vi "Start.vi"(8 "error in (no error)":errorcluster, 11 "TrialBasedExperiment in":refnum<class "TrialBasedExperiment.lvclass">) -> (0 "error out":errorcluster, 3 "TrialBasedExperiment out":refnum<class "TrialBasedExperiment.lvclass">)   [LabVIEW 2010, in "TrialBasedExperiment.lvclass"]
uses:
  TrialBasedExperiment.lvclass
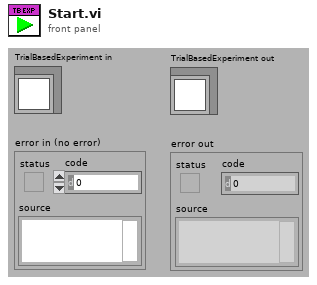
[diagram p1: front panel]
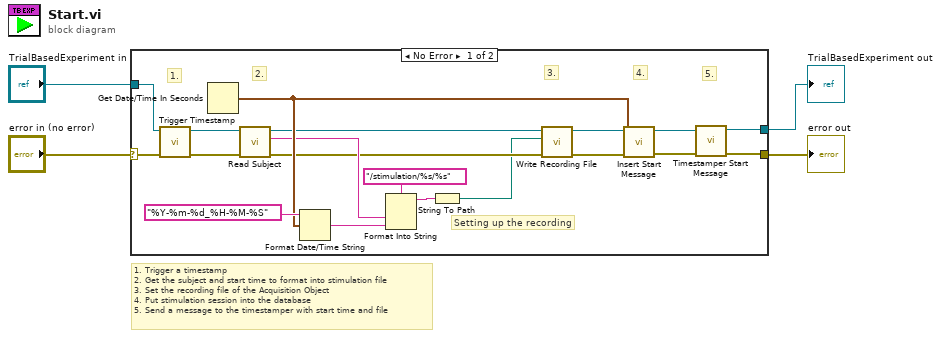
[diagram p0: block diagram]
diagram:
  # "1. Trigger a timestamp\n2. Get the subject and start time to format into stimulation file\n3. Set the recording file of the Acquisition Object\n4. Put stimulation session into the database\n5. Send a message to the timestamper with start time and file"
  n1 = case shown="No Error" "error in (no error)" {
    selector: "error in (no error)" -> [w23 w25]
    tunnel: [w19 w25] -> w3
    tunnel: [w18 w24] -> w1
    tunnel: "TrialBasedExperiment in" -> [w22 w24]
    frame No Error {
      # "5."
      # "4."
      # "3."
      # "2."
      # "1."
      # "Setting up the recording"
      n2 = call-dynamic "Trigger Timestamp.vi"("error in (no error)"=w23, "TrialBasedExperiment in"=w22) -> ("error out"=w12:errorcluster, "TrialBasedExperiment out"=w13:refnum<class "TrialBasedExperiment.lvclass">)  [unwired: 8 in]
      n3 = Get Date/Time In Seconds() -> (seconds since 1Jan1904=w16:timestamp)
      n4 = call-dynamic "Read Subject.vi"("error in (no error)"=w12, "TrialBasedExperiment in"=w13) -> ("error out"=w9:errorcluster, "Subject"=w11:string, "TrialBasedExperiment out"=w10:refnum<class "TrialBasedExperiment.lvclass">)  [unwired: 7 in]
      n5 = Format Date/Time String(time format string (%c)="%Y-%m-%d_%H-%M-%S", seconds (now)=w16) -> (date/time string=w14:string)  [unwired: 1 in]
      n6 = Format Into String(format string="/stimulation/%s/%s", w11, w14) -> (resulting string=w6:string)  [unwired: 2 in, 1 out]
      n7 = String To Path(string=w6) -> (path=w5:path)
      n8 = call-dynamic "Write Recording File.vi"("error in (no error)"=w9, "Recording File"=w5, "AcquistionObject in"=w10) -> ("error out"=w7:errorcluster, "AcquistionObject out"=w8:refnum<class "TrialBasedExperiment.lvclass">)  [unwired: 7 in]
      n9 = call-dynamic "Insert Start Message.vi"("error in (no error)"=w7, "Start Time"=w16, "TrialBasedExperiment in"=w8) -> ("error out"=w20:errorcluster, "TrialBasedExperiment out"=w21:refnum<class "TrialBasedExperiment.lvclass">)  [unwired: 7 in]
      n10 = call-dynamic "Timestamper Start Message.vi"("error in (no error)"=w20, "AcquistionObject in"=w21) -> ("error out"=w19:errorcluster, "AcquistionObject out"=w18:refnum<class "TrialBasedExperiment.lvclass">)  [unwired: 8 in]
    }
    frame Error {
    }
  }
  "error out" <- w3
  "TrialBasedExperiment out" <- w1
